vi "Get SVG Image Size.vi"(3 "error in (no error)":errorcluster, 5 "XML File Path In":path) -> (0 "error out":errorcluster, 1 "Image Size":cluster{"Width":dbl, "Height":dbl}, 2 "XML File Path Out":path)   [LabVIEW 2019]
doc: "This VI gets the SVG image size using XPath and regex."
uses:
  <vilib>/regexp/Match Regular Expression.xnode
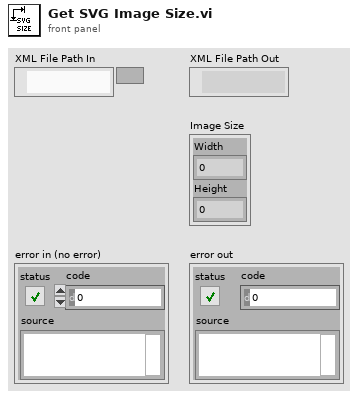
[diagram p1: front panel]
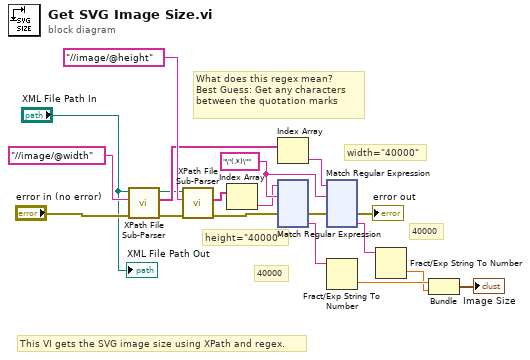
[diagram p0: block diagram]
diagram:
  w8 = "\"(.*)\"" ("search string")
  # "40000"
  # "height=\"40000\""
  # "40000"
  # "width=\"40000\""
  # "What does this regex mean?\nBest Guess: Get any characters between the quotation marks"
  # "This VI gets the SVG image size using XPath and regex."
  n1 = call "XPath File Sub-Parser.vi"("error in (no error)"="error in (no error)", "XPath Expression"="//image/@width" ("XPath expression"), "XML File Path In"="XML File Path In") -> ("error out"=w15:errorcluster, "Array of Results"=w12:string[], "XML File Path Out"=w10:path)  [unwired: 6 in]
  n2 = call "XPath File Sub-Parser.vi"("error in (no error)"=w15, "XPath Expression"="//image/@height" ("XPath expression"), "XML File Path In"=w10) -> ("error out"=w3:errorcluster, "Array of Results"=w13:string[])  [unwired: 6 in, 1 out]
  n3 = Index Array(array=w13) -> (element=w7:string)  [unwired: 1 in]
  n4 = Index Array(array=w12) -> (element=w6:string)  [unwired: 1 in]
  n5 = xnode "Match Regular Expression"("input string"=w7, "regular expression"=w8, "error in"=w3) -> ("error out"=w2:errorcluster, "submatch 1"=w4:string)  [unwired: 3 in, 4 out]
  n6 = xnode "Match Regular Expression"("input string"=w6, "regular expression"=w8, "error in"=w2) -> ("error out"=→"error out":errorcluster, "submatch 1"=w5:string)  [unwired: 3 in, 4 out]
  n7 = Fract/Exp String To Number(string=w4) -> (number=w18:dbl)  [unwired: 3 in, 1 out]
  n8 = Fract/Exp String To Number(string=w5) -> (number=w17:dbl)  [unwired: 3 in, 1 out]
  n9 = Bundle(w18, w17) -> (→"Image Size":cluster{dbl, dbl})  [unwired: 1 in]
  "XML File Path Out" <- "XML File Path In"
